vi "Event Handle Loop_Pop-out Panel_Initialize.vi"(8 "error in (no error)":errorcluster, 10 "VI Refnum":refnum<vi>, 11 "QTab Class in":refnum<class "QTab Class.lvclass">) -> (0 "error out":errorcluster, 3 "QTab Class out":refnum<class "QTab Class.lvclass">)   [LabVIEW 2020, in "QTab.lvlib" / "QTab Class.lvclass"]
uses:
  QTab Class.lvclass
  <vilib>/Utility/miscctls.llb/LVRectTypeDef.ctl
  QTab Class.lvclass/QTab Class.ctl
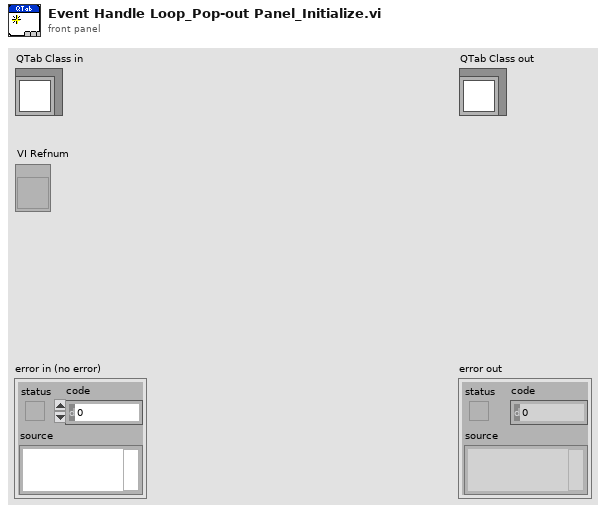
[diagram p1: front panel]
types:
  T1 = enum32{"Invalid", "Standard", "Closed", "Hidden", "Minimized", "Maximized"}
  T2 = typedef "LVRectTypeDef.ctl" = cluster{"Left":i16, "Top":i16, "Right":i16, "Bottom":i16}
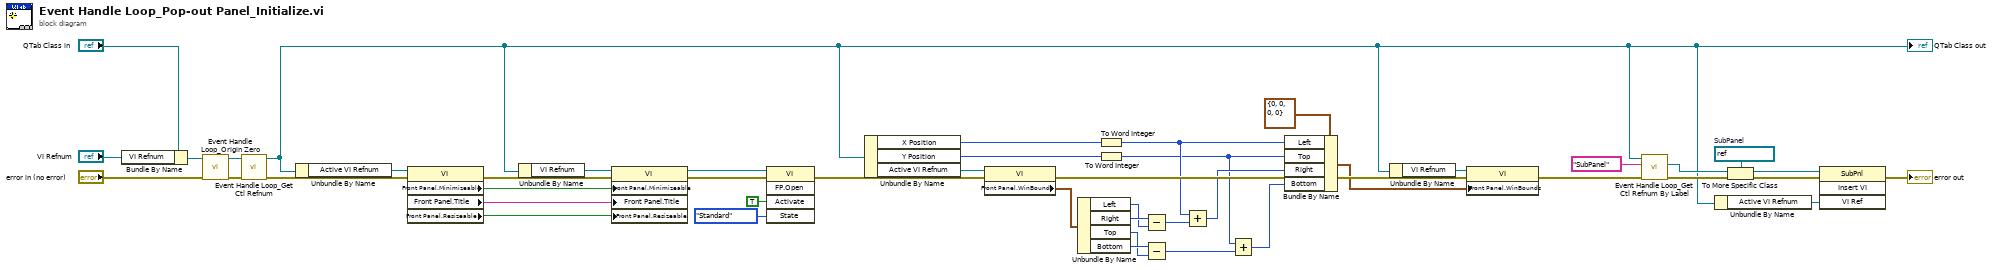
[diagram p0: block diagram]
diagram:
  w14 = refnum<vi> refnum  # SubPanel
  n1 = Bundle By Name(cluster="QTab Class in", "VI Refnum"="VI Refnum") -> (w18:refnum<class "QTab Class.lvclass">)
  n2 = call "Event Handle Loop_Origin Zero.vi"("error in (no error)"="error in (no error)", "QTab Class in"=w18) -> ("error out"=w20:errorcluster, "QTab Class out"=w19:refnum<class "QTab Class.lvclass">)  [unwired: 8 in]
  n3 = call "Event Handle Loop_Get Ctl Refnum.vi"("error in (no error)"=w20, "QTab Class in"=w19) -> ("error out"=w7:errorcluster, "QTab Class out"=w2:refnum<class "QTab Class.lvclass">)  [unwired: 8 in]
  "QTab Class out" <- w2
  n4 = Unbundle By Name(w2) -> ("Active VI Refnum"=w3:refnum<vi>)
  n5 = property class="VI"(reference=w3, error in=w7) -> (error out=w46:errorcluster, "Front Panel.Minimizeable"=w45:bool, "Front Panel.Title"=w44:string, "Front Panel.Resizeable"=w43:bool)  [unwired: 1 out]
  n6 = Unbundle By Name(w2) -> ("VI Refnum"=w1:refnum<vi>)
  n7 = property class="VI"(reference=w1, error in=w46, "Front Panel.Minimizeable"=w45, "Front Panel.Title"=w44, "Front Panel.Resizeable"=w43) -> (reference out=w4:refnum<vi>, error out=w9:errorcluster)
  n8 = invoke class="VI" method="FP.Open"(reference=w4, error in=w9, "Activate"=TRUE ("Activate?"), "State"=T1."Standard") -> (error out=w8:errorcluster)  [unwired: 1 in, 4 out]
  n9 = Unbundle By Name(w2) -> ("X Position"=w34:i16, "Y Position"=w33:i16, "Active VI Refnum"=w26:refnum<vi>)
  n10 = property class="VI"(reference=w26, error in=w8) -> (error out=w36:errorcluster, "Front Panel.WinBounds"=w42:T2)  [unwired: 1 out]
  n11 = Unbundle By Name(w42) -> ("Left"=w40:i16, "Right"=w41:i16, "Top"=w38:i16, "Bottom"=w39:i16)
  n12 = To Word Integer(number=w34) -> (16bit integer=w32:i16)
  n13 = To Word Integer(number=w33) -> (16bit integer=w29:i16)
  n14 = Subtract(x=w41, y=w40) -> (x-y=w37:i16)
  n15 = Subtract(x=w39, y=w38) -> (x-y=w30:i16)
  n16 = Add(x=w32, y=w37) -> (x+y=w31:i16)
  n17 = Add(x=w29, y=w30) -> (x+y=w28:i16)
  n18 = Bundle By Name(cluster=T2 {"Left"=0, "Top"=0, "Right"=0, "Bottom"=0} ("Front Panel Window:Panel Bounds"), "Left"=w32, "Top"=w29, "Right"=w31, "Bottom"=w28) -> (w27:T2)
  n19 = Unbundle By Name(w2) -> ("VI Refnum"=w10:refnum<vi>)
  n20 = property class="VI"(reference=w10, error in=w36, "Front Panel.WinBounds"=w27) -> (error out=w6:errorcluster)  [unwired: 1 out]
  n21 = call "Event Handle Loop_Get Ctl Refnum By Label.vi"("error in (no error)"=w6, "Label"="SubPanel", "QTab Class in"=w2) -> ("error out"=w16:errorcluster, "Ctl Refnum"=w15:refnum<vi>)  [unwired: 6 in, 1 out]
  n22 = Unbundle By Name(w2) -> ("Active VI Refnum"=w11:refnum<vi>)
  n23 = To More Specific Class(target class=w14, reference=w15, error in=w16) -> (specific class reference=w12:refnum<vi>, error out=w13:errorcluster)
  n24 = invoke class="SubPnl" method="Insert VI"(reference=w12, error in=w13, "VI Ref"=w11) -> (error out=→"error out":errorcluster)  [unwired: 1 in, 3 out]
